vi "Volts to dB.vi"(10 "Full scale range":dbl, 11 "Voltage(V)":dbl) -> (3 "Voltage(dB)":dbl)   [LabVIEW 2023]
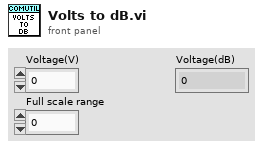
[diagram p1: front panel]
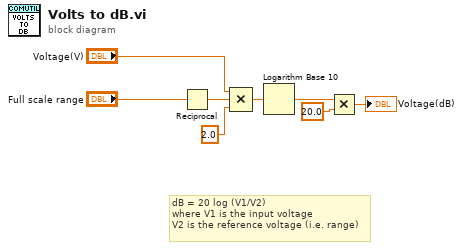
[diagram p0: block diagram]
diagram:
  # "dB = 20 log (V1/V2)\nwhere V1 is the input voltage\nV2 is the reference voltage (i.e. range)"
  n1 = Reciprocal(x="Full scale range") -> (1/x=w3:dbl)
  n2 = Compound Arithmetic op=MULTIPLY("Voltage(V)", w3, 2.0 ("y")) -> (w7:dbl)
  n3 = Logarithm Base 10(1:w7) -> (0:w6:dbl)
  n4 = Multiply(x=w6, y=20.0) -> (x*y=→"Voltage(dB)":dbl)
